vi "ExitApplication Event Callback.vi"(4 "Quit Application Event":refnum<user-event>, 6 "CtlRef":refnum<k7>, 7 "Event common data":cluster{"Source":i32, "Type":u32, "Time":u32}) -> ()   [LabVIEW 2025, in "Config Tool.lvlib"]
doc: "The Application Manager generates the ExitApplication event when TestStand is finished shutting down.\nThis event signals that the operator interface can stop."
uses:
  Config Tool.lvlib
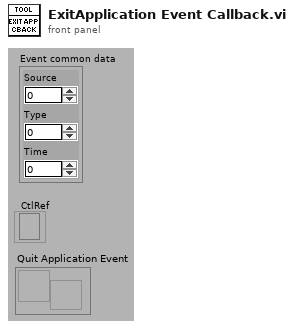
[diagram p1: front panel]
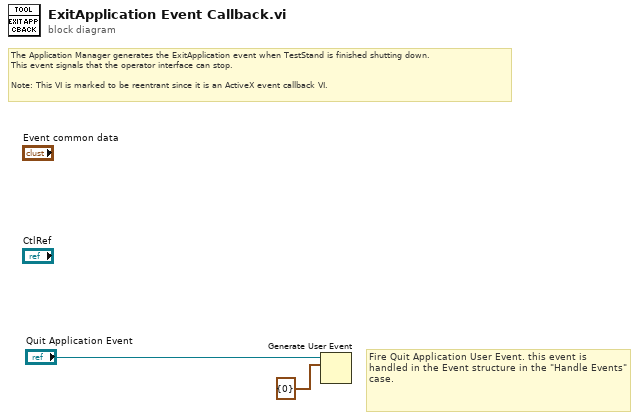
[diagram p0: block diagram]
diagram:
  # "Fire Quit Application User Event. this event is handled in the Event structure in the \"Handle Events\" case."
  # "The Application Manager generates the ExitApplication event when TestStand is finished shutting down.\nThis event signals that the operator interface can stop.\n\nNote: This VI is marked to be reentrant since it is an ActiveX event callback VI."
  n1 = Generate User Event(user event="Quit Application Event", event data cluster=cluster{i32} {0}) -> ()  [unwired: 2 in, 2 out]
